vi "mWmotor_get_stepcount.vi"(8 "error in (no error)":errorcluster, 10 "milliseconds to wait":u32=100, 11 "VISA resource name":refnum<visa-resource-name>) -> (0 "error out":errorcluster, 2 "Revolutions":dbl, 3 "VISA resource name out":refnum<visa-resource-name>)   [LabVIEW 2019]
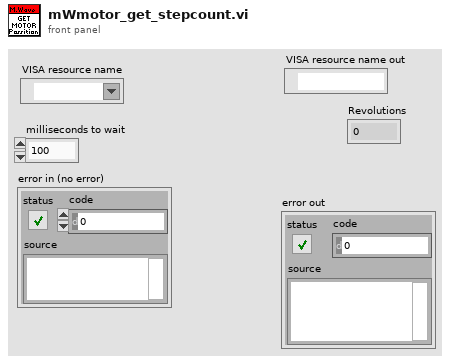
[diagram p1: front panel]
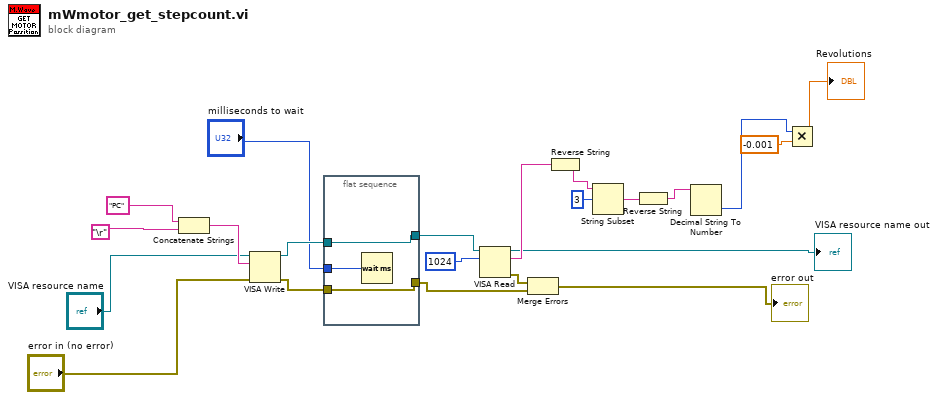
[diagram p0: block diagram]
diagram:
  n1 = Concatenate Strings("PC" ("string"), "\r") -> (w22:string)
  n2 = VISA Write(VISA resource name="VISA resource name", write buffer=w22, error in (no error)="error in (no error)") -> (VISA resource name out=w18:refnum<visa-resource-name>, error out=w19:errorcluster)  [unwired: 1 out]
  n3 = flat-sequence {
    tunnel: [w25] -> w13
    tunnel: w19 -> [w25]
    tunnel: [w24] -> w17
    tunnel: w18 -> [w24]
    tunnel: "milliseconds to wait" -> [w23]
    frame #0 {
      n4 = Wait (ms)(milliseconds to wait=w23) -> ()  [unwired: 1 out]
    }
  }
  n5 = VISA Read(VISA resource name=w17, byte count=u32 1024) -> (VISA resource name out=→"VISA resource name out":refnum<visa-resource-name>, read buffer=w11:string, error out=w12:errorcluster)  [unwired: 1 in, 1 out]
  n6 = Merge Errors(w12, w13) -> (→"error out":errorcluster)
  n7 = Reverse String(1:w11) -> (0:w9:string)
  n8 = String Subset(string=w9, offset (0)=3) -> (substring=w8:string)  [unwired: 1 in]
  n9 = Reverse String(1:w8) -> (0:w7:string)
  n10 = Decimal String To Number(string=w7) -> (number=w1:i32)  [unwired: 2 in, 1 out]
  n11 = Multiply(x=w1, y=-0.001) -> (x*y=→"Revolutions":dbl)
